vi "Circle XY (wSubVI) DegRad.vi"() -> ()   [LabVIEW 2019]
panel:
  in  "Angle Units Selection":enum32{"Degree", "Radians"}(tab)
  out "Angle (in Radians)":dbl
  in  "Angle (Degree)":dbl
  out "Angle (in Degrees)":dbl
  in  "Angle (Radians)":dbl
  out "Circle with XY @ Angle":cluster{dbl[], dbl[]}[](graph)
  out "Y":dbl format="%#.4f"
  out "X":dbl format="%#.4f"
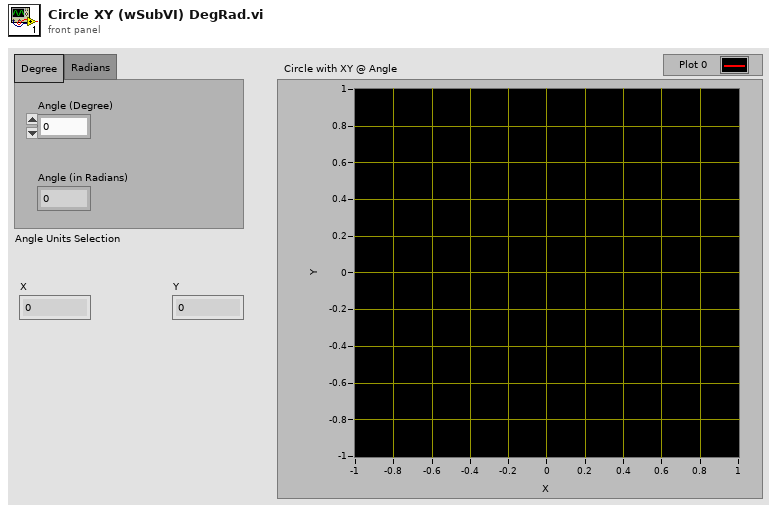
[diagram p1: front panel]
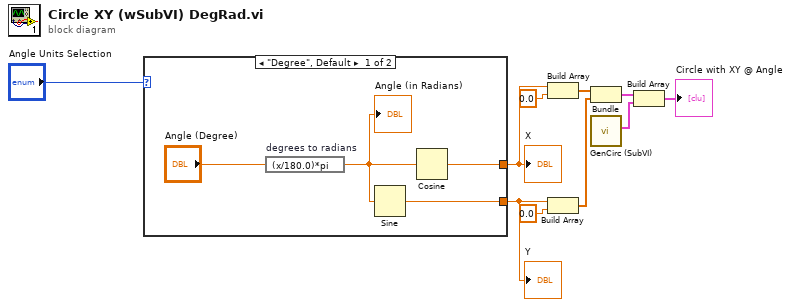
[diagram p0: block diagram]
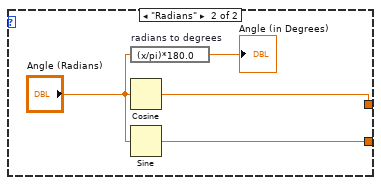
[diagram p2: hidden frame]
diagram:
  n1 = case shown="\"Degree\", Default" "Angle Units Selection" {
    tunnel: [w12 w16] -> w2
    tunnel: [w11 w15] -> w1
    frame "Degree", Default {
      n2 = expression code="(x/180.0)*pi" "degrees to radians"("Angle (Degree)") -> (w13:dbl)
      "Angle (in Radians)" <- w13
      n3 = Sine(x=w13) -> (sin(x)=w11:dbl)
      n4 = Cosine(x=w13) -> (cos(x)=w12:dbl)
    }
    frame "Radians" {
      n5 = expression code="(x/pi)*180.0" "radians to degrees"("Angle (Radians)") -> (→"Angle (in Degrees)":dbl)
      n6 = Cosine(x="Angle (Radians)") -> (cos(x)=w16:dbl)
      n7 = Sine(x="Angle (Radians)") -> (sin(x)=w15:dbl)
    }
  }
  "X" <- w2
  "Y" <- w1
  n8 = Build Array(w2, 0.0) -> (w10:dbl[])
  n9 = Build Array(w1, 0.0) -> (w9:dbl[])
  n10 = Bundle(w10, w9) -> (w6:cluster{dbl[], dbl[]})  [unwired: 1 in]
  n11 = call "GenCirc (SubVI).vi"() -> ("Cluster"=w5:cluster{dbl[], dbl[]})  [unwired: 11 in]
  n12 = Build Array(w6, w5) -> (→"Circle with XY @ Angle":cluster{dbl[], dbl[]}[])
